vi "Build Daily VI Package_vipm_lvcicd.vi"(8 "error in (no error)":errorcluster, 9 "LabVIEW Version":string="19.0", 10 "vipb":path) -> (0 "error out":errorcluster, 2 "Build Output":path, 4 "New VI Package Build Spec Data":T1, 6 "Pre VI Package Build Spec Data":T1)   [LabVIEW 2014]
uses:
  <vilib>/JKI/VIPM API/command-line/support/VI Package Build Spec Data Cluster_vipm_api.ctl
  <vilib>/JKI/VIPM API/command-line/support/Version Info Cluster_vipm_api.ctl
  <vilib>/JKI/VIPM API/VIPM API_vipm_api.lvlib
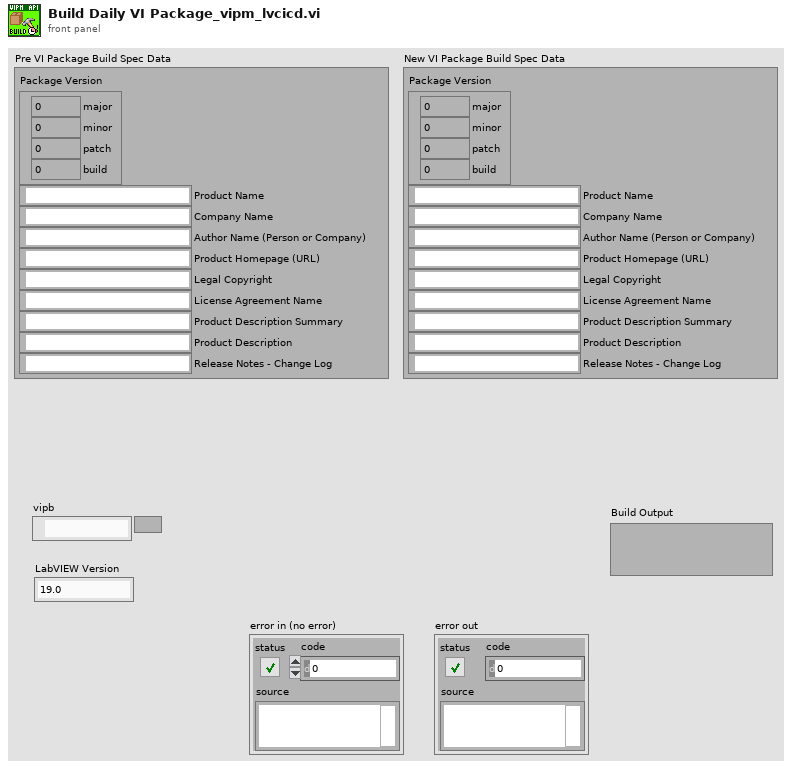
[diagram p1: front panel]
types:
  T1 = typedef "VIPM API_vipm_api.lvlib/VI Package Build Spec Data Cluster_vipm_api.ctl" = cluster{"Package Version":T2, "Product Name":string, "Company Name":string, "Author Name (Person or Company)":string, "Product Homepage (URL)":string, "Legal Copyright":string, "License Agreement Name":string, "Product Description Summary":string, "Product Description":string, "Release Notes - Change Log":string}
  T2 = typedef "VIPM API_vipm_api.lvlib/Version Info Cluster_vipm_api.ctl" = cluster{"major":u32, "minor":u32, "patch":u32, "build":u32}
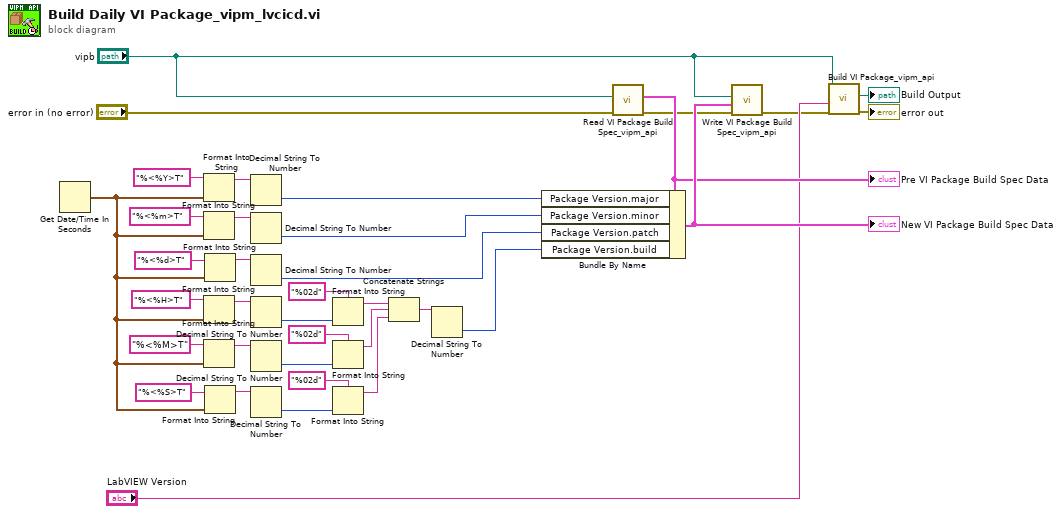
[diagram p0: block diagram]
diagram:
  n1 = Get Date/Time In Seconds() -> (seconds since 1Jan1904=w15:timestamp)
  n2 = Format Into String(format string="%<%Y>T", w15) -> (resulting string=w27:string)  [unwired: 2 in, 1 out]
  n3 = Format Into String(format string="%<%m>T", w15) -> (resulting string=w29:string)  [unwired: 2 in, 1 out]
  n4 = Format Into String(format string="%<%H>T", w15) -> (resulting string=w10:string)  [unwired: 2 in, 1 out]
  n5 = Format Into String(format string="%<%M>T", w15) -> (resulting string=w11:string)  [unwired: 2 in, 1 out]
  n6 = Format Into String(format string="%<%d>T", w15) -> (resulting string=w32:string)  [unwired: 2 in, 1 out]
  n7 = Format Into String(format string="%<%S>T", w15) -> (resulting string=w12:string)  [unwired: 2 in, 1 out]
  n8 = Decimal String To Number(string=w27) -> (number=w28:i32)  [unwired: 2 in, 1 out]
  n9 = Decimal String To Number(string=w29) -> (number=w33:i32)  [unwired: 2 in, 1 out]
  n10 = Decimal String To Number(string=w32) -> (number=w34:i32)  [unwired: 2 in, 1 out]
  n11 = Decimal String To Number(string=w10) -> (number=w9:i32)  [unwired: 2 in, 1 out]
  n12 = Decimal String To Number(string=w11) -> (number=w6:i32)  [unwired: 2 in, 1 out]
  n13 = Decimal String To Number(string=w12) -> (number=w4:i32)  [unwired: 2 in, 1 out]
  n14 = Format Into String(format string="%02d", w9) -> (resulting string=w3:string)  [unwired: 2 in, 1 out]
  n15 = Format Into String(format string="%02d", w6) -> (resulting string=w2:string)  [unwired: 2 in, 1 out]
  n16 = Format Into String(format string="%02d", w4) -> (resulting string=w1:string)  [unwired: 2 in, 1 out]
  n17 = Concatenate Strings(w3, w2, w1) -> (w14:string)
  n18 = Decimal String To Number(string=w14) -> (number=w13:i32)  [unwired: 2 in, 1 out]
  n19 = call <vilib>:"Read VI Package Build Spec_vipm_api.vi"("error in (no error)"="error in (no error)", "Path to VIPB File"="vipb") -> ("error out"=w24:errorcluster, "VI Package Build Spec Data"=w25:T1)  [unwired: 8 in]
  "Pre VI Package Build Spec Data" <- w25
  n20 = Bundle By Name(cluster=w25, "Package Version.major"=w28, "Package Version.minor"=w33, "Package Version.patch"=w34, "Package Version.build"=w13) -> (w35:T1)
  "New VI Package Build Spec Data" <- w35
  n21 = call <vilib>:"Write VI Package Build Spec_vipm_api.vi"("error in (no error)"=w24, "VI Package Build Spec Data"=w35, "Path to VIPB File"="vipb") -> ("error out"=w22:errorcluster)  [unwired: 8 in]
  n22 = call <vilib>:"Build VI Package_vipm_api.vi"("error in (no error)"=w22, "LabVIEW Version"="LabVIEW Version", "Path to VIPB File"="vipb") -> ("error out"=→"error out":errorcluster, "Build Output"=→"Build Output":path)  [unwired: 7 in]
